vi "niFpgaPID_PDMemoryRead.vi"(1 "channel (0)":u8) -> (4 "data memory out":refnum<k21>="Data", 6 "manual memory out":refnum<k21>="Manual", 14 "parameters out":T1, 15 "state out":T2)   [LabVIEW 2020]
uses:
  <vilib>/rvi/Analysis/control/PID/Typedef/niFpgaPID_PDState.ctl
  <vilib>/rvi/Analysis/control/PID/Typedef/niFpgaPID_PDParameters.ctl
  <vilib>/Platform/TimedLoop/XDataNode/timing_clust.ctl
  <vilib>/Platform/TimedLoop/XDataNode/nitl_modes.ctl
  <vilib>/Platform/TimedLoop/XDataNode/wakeup.ctl
  <vilib>/rvi/Emulation/niFpgaSctlEmulationGetInTimedLoop.vi
  <vilib>/Utility/error.llb/Clear Errors.vi
  <vilib>/rvi/DataTransferAndStorage/Container/Common/niFpgaContainerGetUniqueNameForEmu.vi
  <vilib>/rvi/DataTransferAndStorage/Container/Common/niFpgaContainerSetEmuInfo.vi
  <vilib>/rvi/eio/common/nirviEmuReportErrorAndStop.vi
  <vilib>/rvi/DataTransferAndStorage/Container/Common/niFpgaContainerExecOnDevCompGetState.vi
  <vilib>/rvi/Emulation/niFpgaEmulationIsFPGAContextNoSignature.vi
  <vilib>/rvi/Emulation/niFpgaProcessEmulError.vi
  <vilib>/rvi/errors/nirviReportUnexpectedCaseInternalError (U32).vi
  <vilib>/rvi/Memory/Memory_Emulation/niFpgaMemoryEmulationCacheClearOnFirstRun.vi
  <vilib>/rvi/Memory/Memory_Emulation/nirvimemoryEmulationManagerCache_MakeExclusive.vi
  <vilib>/rvi/Memory/Memory_Emulation/niFpgaMemoryEmulationValidateCache.vi
  <vilib>/rvi/Memory/Memory_Emulation/nirvimemoryEmulationManagerCache_InsertValue.vi
  <vilib>/rvi/Memory/Memory_Emulation/nirvimemoryEmulationManagerCache_ReleaseExclusive.vi
  <vilib>/rvi/Memory/Memory_Emulation/nirvimemoryEmulationManagerCache_GetValue.vi
  <vilib>/rvi/Memory/Memory_Emulation/nirvimemoryEmulationManagerCache_SetValue.vi
  <vilib>/rvi/Emulation/niFpgaSctlEmulationResourceMgr.vi
  <vilib>/Platform/TimedLoop/XDataNode/XDataNode.xnode
  <vilib>/rvi/LocalResourceManager/LocalResourceManager.xnode
  <vilib>/rvi/DataTransferAndStorage/Container/XNode/niFpgaContainer.xnode
  <vilib>/rvi/Memory/Memory_Emulation/niFpgaMemoryEmulationRefIn.vi
  <vilib>/Platform/TimedLoop/XDataNode/XDNodeRunTimeDep.lvlib
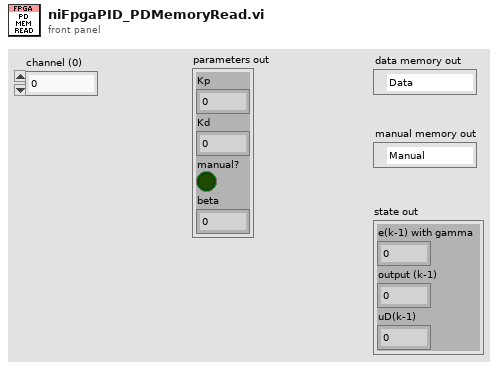
[diagram p1: front panel]
types:
  T1 = typedef "niFpgaPID_PDParameters.ctl" = cluster{"Kp":sgl, "Kd":sgl, "manual?":bool, "beta":sgl}
  T2 = typedef "niFpgaPID_PDState.ctl" = cluster{"e(k-1) with gamma":sgl, "output (k-1)":sgl, "uD(k-1)":sgl}
  T3 = typedef "XDNodeRunTimeDep.lvlib/timing_clust.ctl" = cluster{"Expected End [f-1]":u64, "Actual End [f-1]":u64, "Finished Late? [f-1]":bool, "Expected End [i-1]":u64, "Actual End [i-1]":u64, "Finished Late? [i-1]":bool, "Expected Start [i]":u64, "Actual Start [i]":u64, "Expected Start [f]":u64, "Actual Start [f]":u64, "Source Name":string, "Structure Name":string, "Period":i64, "Deadline":i64, "Offset":i64, "Start":i64, "Priority":i32, "Timeout":i32, "Mode":T4, "Wakeup Reason":T5, "Error":errorcluster, "Source Type":string, "Secondary Source Type":string, "Global End Time":u64, "Global Start Time":u64, "Frame Duration":u64, "Iteration Duration":u64, "Assigned CPU":i32, "I/O Scan Engine Mode":u32}
  T4 = typedef "XDNodeRunTimeDep.lvlib/nitl_modes.ctl" = enum32{"No Change", "Process missed periods, maintain original phase", "Discard missed periods, maintain original phase", "Process missed periods, ignore original phase", "Discard missed periods, ignore original phase"}
  T5 = typedef "XDNodeRunTimeDep.lvlib/wakeup.ctl" = enum32{"Normal", "Aborted", "Asynchronous wakeup", "Timing source error", "Timed loop error", "Timeout"}
  T6 = cluster{"data 1":sgl, "data 2":sgl, "data 3":sgl}
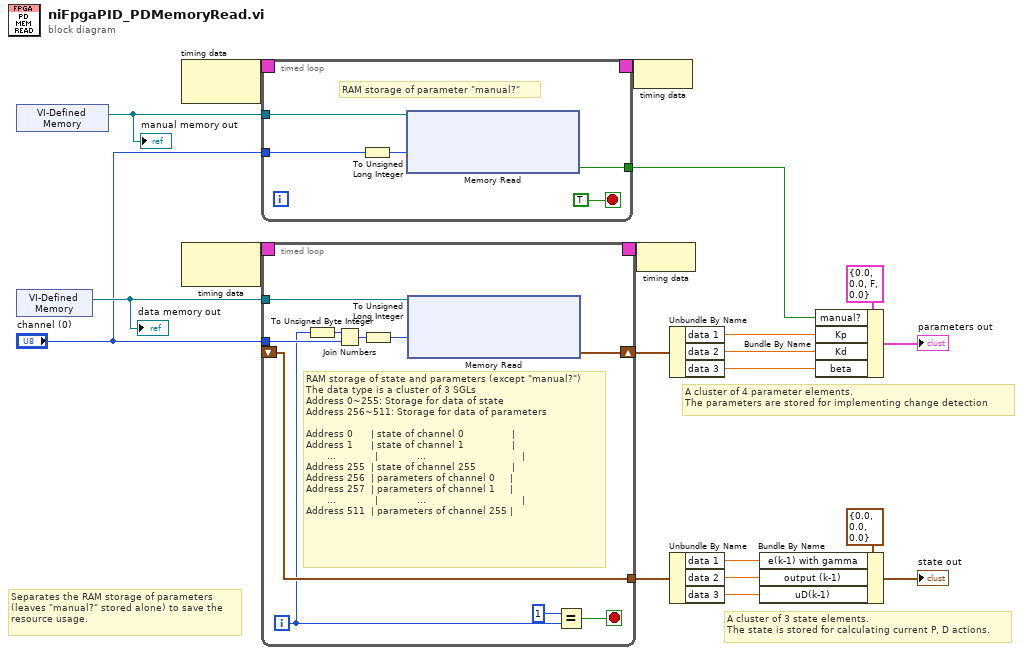
[diagram p0: block diagram]
diagram:
  # "Separates the RAM storage of parameters\n(leaves \"manual?\" stored alone) to save the \nresource usage."
  # "A cluster of 4 parameter elements.\nThe parameters are stored for implementing change detection"
  # "A cluster of 3 state elements.\nThe state is stored for calculating current P, D actions."
  n1 = xnode "VI-Defined Memory"() -> ("Memory Out"=w2:refnum<k21>)
  "manual memory out" <- w2
  n2 = xnode "VI-Defined Memory"() -> ("Memory Out"=w11:refnum<k21>)
  "data memory out" <- w11
  n3 = node-c288() -> (w9:T3)  [unwired: 1 in]
  n4 = node-c288() -> (w20:T3)  [unwired: 1 in]
  n5 = timed-loop {
    timing: w9 -> [_]
    timing-out: [_] -> w8
    tunnel: w2 -> [w23]
    tunnel: [w21] -> w6
    tunnel: "channel (0)" -> [w25]
    stop <- TRUE stop-if-true
    # "RAM storage of parameter \"manual?\""
    n6 = To Unsigned Long Integer(number=w25) -> (unsigned 32bit integer=w22:u32)
    n7 = xnode "Memory Read"("Address"=w22, "Memory In"=w23) -> ("Data"=w21:bool)  [unwired: 1 out]
  }
  n8 = timed-loop {
    tunnel: "channel (0)" -> [w36]
    timing: w20 -> [_]
    timing-out: [_] -> w19
    tunnel: w11 -> [w30]
    shift-right: [w28] -> w18
    shift-left: _ -> [w37]
    tunnel: [w37] -> w17
    i -> [w33]
    stop <- w34 stop-if-true
    # "RAM storage of state and parameters (except \"manual?\")\nThe data type is a cluster of 3 SGLs \nAddress 0~255: Storage for data of state\nAddress 256~511: Storage for data of parameters\n                                                                         \nAddress 0      | state of channel 0                | \nAddress 1      | state of channel 1                | \n       ...             |             ...                                |\nAddress 255  | state of channel 255            | \nAddress 256  | parameters of channel 0     | \nAddress 257  | parameters of channel 1     | \n       ...             |             ...                                |\nAddress 511  | parameters of channel 255 |"
    n9 = To Unsigned Byte Integer(number=w33) -> (unsigned 8bit integer=w32:u8)
    n10 = Join Numbers(hi=w32, lo=w36) -> ((hi.lo)=w35:u16)
    n11 = To Unsigned Long Integer(number=w35) -> (unsigned 32bit integer=w29:u32)
    n12 = xnode "Memory Read"("Address"=w29, "Memory In"=w30) -> ("Data"=w28:T6)  [unwired: 1 out]
    n13 = Equal?(x=1, y=w33) -> (x = y?=w34:bool)
  }
  n14 = node-c288(w8) -> ()
  n15 = node-c288(w19) -> ()
  n16 = Unbundle By Name(w18) -> ("data 1"=w16:sgl, "data 2"=w15:sgl, "data 3"=w10:sgl)
  n17 = Unbundle By Name(w17) -> ("data 1"=w12:sgl, "data 2"=w13:sgl, "data 3"=w14:sgl)
  n18 = Bundle By Name(cluster=T2 {"e(k-1) with gamma"=0.0, "output (k-1)"=0.0, "uD(k-1)"=0.0} ("state"), "e(k-1) with gamma"=w12, "output (k-1)"=w13, "uD(k-1)"=w14) -> (→"state out":T2)
  n19 = Bundle By Name(cluster=T1 {"Kp"=0.0, "Kd"=0.0, "manual?"=FALSE, "beta"=0.0} ("parameters"), "manual?"=w6, "Kp"=w16, "Kd"=w15, "beta"=w10) -> (→"parameters out":T1)
